vi "Process Collision.vi"(11 "Ball-Ball in":refnum<class "Ball-Ball.lvclass">) -> (3 "Ball-Ball out":refnum<class "Ball-Ball.lvclass">)   [LabVIEW 2021, in "Ball-Ball.lvclass"]
doc: "MIT Licence\nCopyright (c) 2024 David Grollier"
uses:
  Ball-Ball.lvclass
  C:/Users/David/Documents/GameSoccerSpace/Source/Collision/Collision.lvclass
  Game Componants/Game Board Component/Movable/Movable.lvclass
  C:/Users/David/Documents/GameSoccerSpace/Source/Game Componants/Game Board Component/Game Board Component.lvclass
  Game Componants/Game Board Component/Movable/Movable.lvclass/Movable.ctl
  Collision.lvclass/Collision.ctl
  <vilib>/Analysis/_algsub.llb/Vector Norm.vi
  <vilib>/Analysis/_algsub.llb/Real Vector Norm.vi
  Collision.lvclass
  Utils/Utils.lvlib
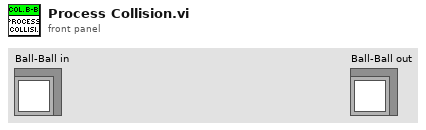
[diagram p1: front panel]
types:
  T1 = typedef "Coordinates.ctl" = cluster{"x":dbl, "y":dbl}
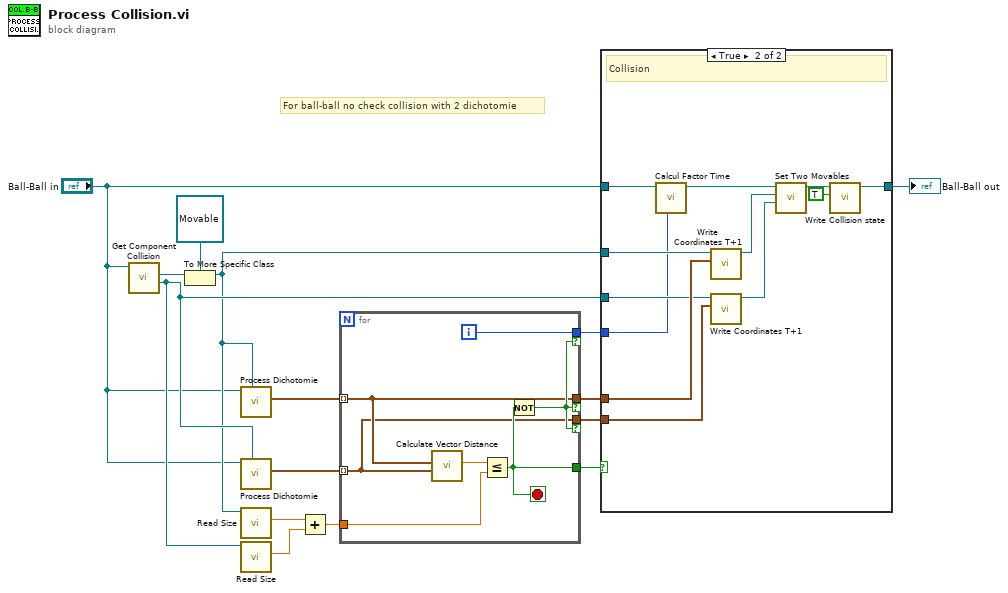
[diagram p0: block diagram]
diagram:
  # "For ball-ball no check collision with 2 dichotomie"
  n1 = call "Get Component Collision.vi"("Collision in"="Ball-Ball in") -> ("Movable out"=w6:refnum<class "Movable.lvclass">, "GB Component out"=w14:refnum<class "Game Board Component.lvclass">)  [unwired: 9 in]
  n2 = To More Specific Class(target class=refnum<class "Movable.lvclass"> refnum ("Movable out"), reference=w14) -> (specific class reference=w4:refnum<class "Movable.lvclass">)  [unwired: 1 in, 1 out]
  n3 = call "Process Dichotomie.vi"("Movable in"=w4, "Collision in"="Ball-Ball in") -> ("Coordinates with dichotomie[] out"=w5:T1[])  [unwired: 8 in, 1 out]
  n4 = call "Process Dichotomie.vi"("Movable in"=w6, "Collision in"="Ball-Ball in") -> ("Coordinates with dichotomie[] out"=w3:T1[])  [unwired: 8 in, 1 out]
  n5 = call "Read Size.vi"("Movable in"=w4) -> ("Size"=w9:dbl)  [unwired: 10 in]
  n6 = call "Read Size.vi"("Movable in"=w6) -> ("Size"=w10:dbl)  [unwired: 10 in]
  n7 = Add(x=w9, y=w10) -> (x+y=w8:dbl)
  n8 = for {
    tunnel: w8 -> [w22]
    tunnel: w5 -> [w18] mode=indexing
    tunnel: w3 -> [w17] mode=indexing
    tunnel: [w19] -> w13 if=w20
    tunnel: [w18] -> w12 if=w20
    tunnel: [w17] -> w11 if=w20
    tunnel: [w21] -> w1
    i -> [w19]
    stop <- w21 stop-if-true
    n9 = call "Calculate Vector Distance.vi"("V2"=w17, "V1"=w18) -> ("Distance out"=w16:dbl)  [unwired: 9 in]
    n10 = Less Or Equal?(x=w16, y=w22) -> (x <= y?=w21:bool)
    n11 = Not(x=w21) -> (.not. x?=w20:bool)
  }
  n12 = case shown="True" w1 {
    tunnel: w13 -> [_ w26]
    tunnel: w12 -> [_ w35]
    tunnel: w11 -> [_ w34]
    tunnel: [w23 w25] -> w7
    tunnel: w4 -> [_ w32]
    tunnel: w6 -> [_ w31]
    tunnel: "Ball-Ball in" -> [w23 w28]
    frame False {
      # "Does nothing"
      # "No collision"
    }
    frame True {
      # "Collision"
      n13 = call "Calcul Factor Time.vi"("Accurate Iteration in"=w26, "Collision in"=w28) -> ("Collision out"=w27:refnum<class "Ball-Ball.lvclass">)  [unwired: 9 in]
      n14 = call "Write Coordinates T+1.vi"("Coordinates"=w35, "Movable in"=w32) -> ("Movable out"=w30:refnum<class "Movable.lvclass">)  [unwired: 9 in]
      n15 = call "Write Coordinates T+1.vi"("Coordinates"=w34, "Movable in"=w31) -> ("Movable out"=w29:refnum<class "Movable.lvclass">)  [unwired: 9 in]
      n16 = call "Set Two Movables.vi"("Movable 2 in"=w29, "Movable 1 in"=w30, "Collision in"=w27) -> ("Collision out"=w33:refnum<class "Ball-Ball.lvclass">)  [unwired: 8 in]
      n17 = call "Write Collision state.vi"("Collision state"=TRUE, "Collision in"=w33) -> ("Collision out"=w25:refnum<class "Ball-Ball.lvclass">)  [unwired: 9 in]
    }
  }
  "Ball-Ball out" <- w7
